vi "stop.vi"(7 "Description":string, 8 "Command Info In":T1, 11 "Synchronication":enum16{"Start", "Wait"}(ring)) -> (0 "Command Info Out":T1)   [LabVIEW 2016]
uses:
  <vilib>/Rock Robotics/WPI/Framework/Command Status Info.ctl
  <vilib>/Rock Robotics/WPI/Framework/Completion Status.ctl
  <vilib>/Rock Robotics/WPI/Framework/Completion Notifier.ctl
  Implementation/Shooter Setpoints.ctl
  Implementation/Shooter Operations.ctl
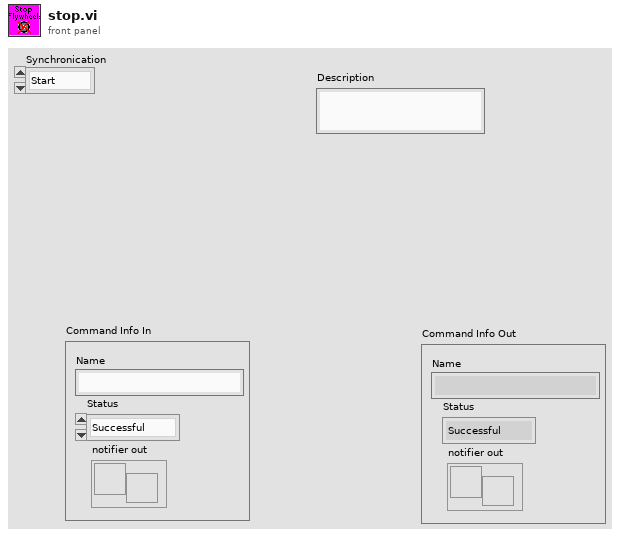
[diagram p1: front panel]
types:
  T1 = typedef "Command Status Info.ctl" = cluster{"Name":string, "Status":T2, "notifier out":T3}
  T2 = typedef "Completion Status.ctl" = enum16{"Successful", "Aborted", "Incomplete"}
  T3 = typedef "Completion Notifier.ctl" = refnum<notifier>
  T4 = typedef "Shooter Setpoints.ctl" = cluster{"Operation":T5, "Setpoint":dbl, "Hood Angle":dbl, "Speed (RPM)":dbl}
  T5 = typedef "Shooter Operations.ctl" = enum16{"Reserve", "Read Current", "Immediate", "Spin Flywheels", "Angle Hood", "Stop flywheels"}
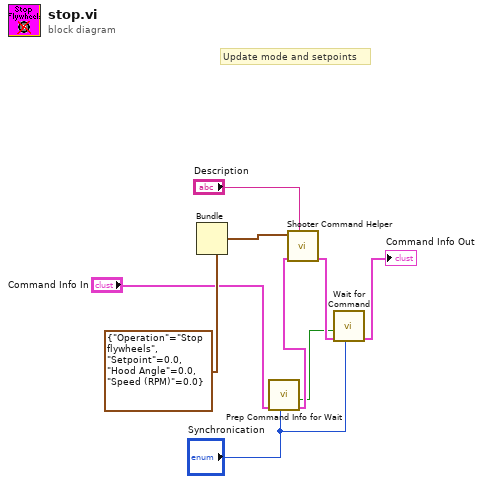
[diagram p0: block diagram]
diagram:
  # "Update mode and setpoints"
  n1 = Bundle(cluster=T4 {"Operation"=enum."Stop flywheels", "Setpoint"=0.0, "Hood Angle"=0.0, "Speed (RPM)"=0.0} ("SubSystem Data")) -> (w7:T4)  [unwired: 4 in]
  n2 = call <vilib>:"Prep Command Info for Wait.vi"("Synchronication"="Synchronication", "Command Info"="Command Info In") -> ("Command Info"=w5:T1, "Allocated"=w2:bool)  [unwired: 8 in]
  n3 = call "Shooter Command Helper.vi"("Description"="Description", "Command Info In"=w5, "SubSystem Data"=w7) -> ("Command Info Out"=w4:T1)  [unwired: 7 in, 1 out]
  n4 = call <vilib>:"Wait for Command.vi"("Synchronication"="Synchronication", "Command Info in"=w4, "Allocated"=w2) -> ("Command Info out"=→"Command Info Out":T1)  [unwired: 8 in]
